vi "Check file size.vi"(8 "error in (no error)":errorcluster, 10 "min size (KB)":i64, 11 "DAQOrcaFlash in":refnum<class "DAQOrcaFlash.lvclass">) -> (0 "error out":errorcluster, 2 "too small?":bool, 3 "DAQOrcaFlash out":refnum<class "DAQOrcaFlash.lvclass">)   [LabVIEW 2012, in "DAQOrcaFlash.lvclass"]
uses:
  DAQOrcaFlash.lvclass
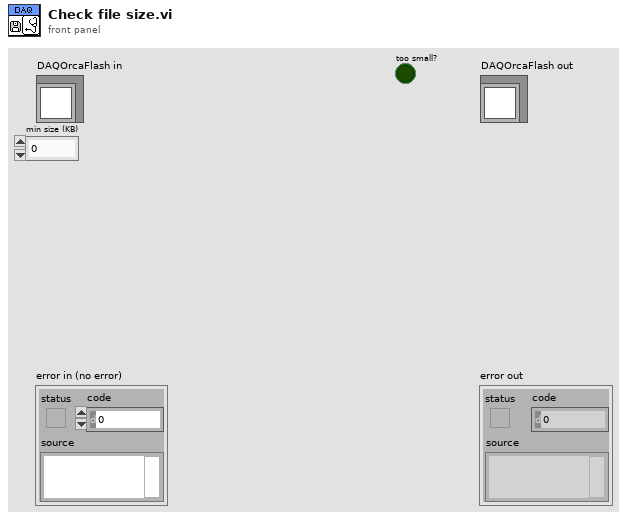
[diagram p1: front panel]
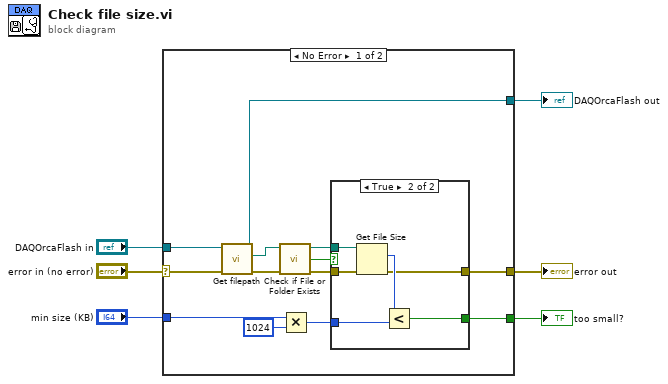
[diagram p0: block diagram]
diagram:
  n1 = case shown="No Error" "error in (no error)" {
    selector: "error in (no error)" -> [w14 w28]
    tunnel: [w15 w28] -> w5
    tunnel: [w13 w27] -> w3
    tunnel: "DAQOrcaFlash in" -> [w12 w27]
    tunnel: "min size (KB)" -> [w18 _]
    tunnel: [w16 _] -> w1
    frame No Error {
      n2 = call "Get filepath.vi"("error in (no error)"=w14, "DAQOrcaFlash in"=w12) -> ("error out"=w9:errorcluster, "full storage path"=w11:path, "DAQOrcaFlash out"=w13:refnum<class "DAQOrcaFlash.lvclass">)  [unwired: 7 in]
      n3 = call <vilib>:"Check if File or Folder Exists.vi"("error in (no error)"=w9, "path"=w11) -> ("error out"=w8:errorcluster, "file or folder exists?"=w7:bool, "dup path"=w10:path)  [unwired: 7 in]
      n4 = Multiply(x=w18, y=i64 1024 ("size (in bytes)")) -> (x*y=w17:i64)
      n5 = case shown="True" w7 {
        tunnel: w17 -> [_ w25]
        tunnel: [_ w24] -> w16
        tunnel: [w20 w23] -> w15
        tunnel: w10 -> [_ w22]
        tunnel: w8 -> [w20 w21]
        frame False {
        }
        frame True {
          n6 = Get File Size(file=w22, error in=w21) -> (size (in bytes)=w26:i64, 0:w23:errorcluster)  [unwired: 1 out]
          n7 = Less?(x=w26, y=w25) -> (x < y?=w24:bool)
        }
      }
    }
    frame Error {
    }
  }
  "error out" <- w5
  "DAQOrcaFlash out" <- w3
  "too small?" <- w1
